vi "Install Template.vi"(8 "error in":errorcluster, 11 "HTML Help Word Template":path) -> (0 "error out":errorcluster)   [LabVIEW 2015, in "HTML Help File Tools.lvlib"]
uses:
  HTML Help File Tools.lvlib
  <vilib>/Utility/sysdir.llb/System Directory Type.ctl
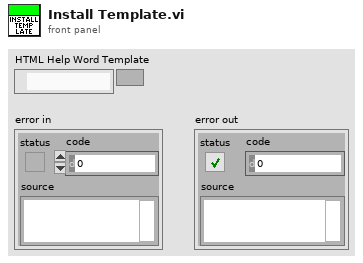
[diagram p1: front panel]
types:
  T1 = typedef "System Directory Type.ctl" = i32
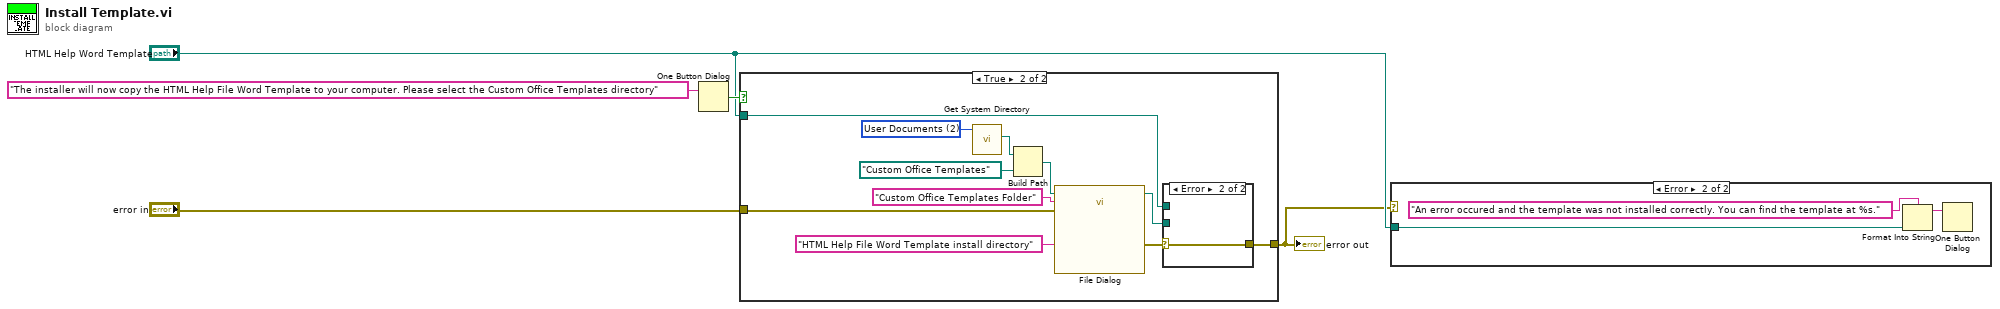
[diagram p0: block diagram]
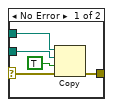
[diagram p4: hidden frame]
diagram:
  n1 = One Button Dialog(message="The installer will now copy the HTML Help File Word Template to your computer. Please select the Custom Office Templates directory") -> (true=w3:bool)  [unwired: 1 in]
  n2 = case shown="True" w3 {
    tunnel: "HTML Help Word Template" -> [_ w9]
    tunnel: "error in" -> [w6 w8]
    tunnel: [w6 w7] -> w1
    frame False {
    }
    frame True {
      w17 = T1 2 items=["User Home"=0, "User Desktop"=1, "User Documents"=2, "User Application Data"=3, "User Preferences"=4, "User Temporary"=5, "Public Documents"=6, "Public Application Data"=7, "Public Preferences"=8, "Public Cache"=13, "System Core Libraries"=9, "System Installed Libraries"=10, "Application Files"=11, "Boot Volume Root"=12] ("system directory type")
      n3 = call <vilib>:"Get System Directory.vi"("system directory type"=w17) -> ("system directory"=w16:path)  [unwired: 10 in]
      n4 = Build Path(base path=w16, name or relative path=path "Custom Office Templates" ("start path")) -> (appended path=w14:path)
      n5 = call "File Dialog"("start path"=w14, "prompt"="HTML Help File Word Template install directory", "default name"="Custom Office Templates Folder", "error in"=w8) -> ("selected path"=w10:path, "error out"=w11:errorcluster)  [unwired: 8 in, 2 out]
      n6 = case shown="Error" w11 {
        selector: w11 -> [w19 w23]
        tunnel: w10 -> [w21 _]
        tunnel: w9 -> [w22 _]
        tunnel: [w18 w23] -> w7
        frame No Error {
          n7 = Copy(8:w19, 9:TRUE ("overwrite (F)"), 10:w21, 11:w22) -> (0:w18:errorcluster)  [unwired: 1 in, 2 out]
        }
        frame Error {
        }
      }
    }
  }
  "error out" <- w1
  n8 = case shown="Error" w1 {
    tunnel: "HTML Help Word Template" -> [_ w26]
    frame No Error {
    }
    frame Error {
      n9 = Format Into String(format string="An error occured and the template was not installed correctly. You can find the template at %s." ("message"), w26) -> (resulting string=w25:string)  [unwired: 2 in, 1 out]
      n10 = One Button Dialog(message=w25) -> ()  [unwired: 1 in, 1 out]
    }
  }
